vi "Eval_SglVar_SglRes.vi"(8 "error in (no error)":errorcluster, 9 "varValue":dbl format="%#_13g", 11 "mupExpr in":refnum<data-value>) -> (0 "error out":errorcluster, 2 "Result":dbl, 3 "mupExpr out":refnum<data-value>)   [LabVIEW 2015, in "mupExpr.lvclass"]
doc: "Updates the value of the selected single variable then evaluates the expression.\nReturns a single result.\n\nIf multiple expressions have been input, the result of the last one in the list is returned.\n\nIf the variables are defined for bulk mode evaluation, only the first set (index 0) will be evaluated."
uses:
  mupExpr.lvclass
  mupExpr.lvclass/mupExpr.ctl
  mupLib/mupCheckError.vi
  mupLib/mupLibPath.vi
  <vilib>/Utility/error.llb/Error Cluster From Error Code.vi
  mupLib/mupLib.lvlib
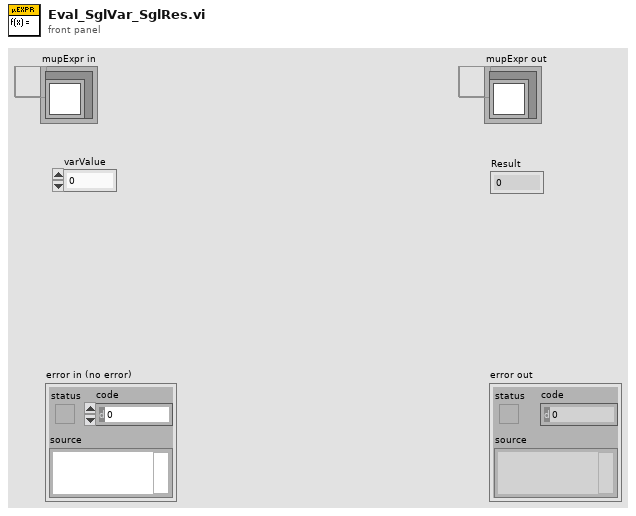
[diagram p1: front panel]
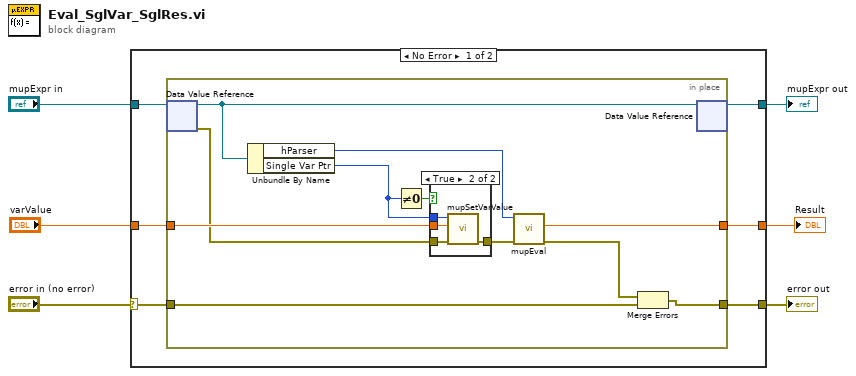
[diagram p0: block diagram]
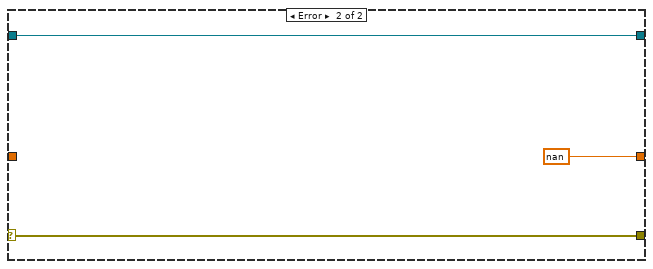
[diagram p3: hidden frame]
diagram:
  n1 = case shown="No Error" "error in (no error)" {
    selector: "error in (no error)" -> [w12 w31]
    tunnel: [w10 w31] -> w5
    tunnel: [w7 w30] -> w3
    tunnel: "mupExpr in" -> [w8 w30]
    tunnel: "varValue" -> [w11 _]
    tunnel: [w9 nan ("Result")] -> w1
    frame No Error {
      n2 = in-place {
        in-place-border: w12 -> [w17]
        in-place-border: w11 -> [w22]
        in-place-border: [w15] -> w10
        in-place-border: [w21] -> w9
        n3 = in-place-dvr #1(w8) -> (w18:refnum<class "mupExpr.lvclass">, w19:errorcluster)
        n4 = Unbundle By Name(w18) -> ("hParser"=w20:u64, "Single Var Ptr"=w23:u64)
        n5 = Not Equal To 0?(x=w23) -> (x != 0?=w13:bool)
        n6 = case shown="True" w13 {
          tunnel: w19 -> [w24 w28]
          tunnel: w22 -> [_ w27]
          tunnel: [w24 w26] -> w14
          tunnel: w23 -> [_ w25]
          frame False {
          }
          frame True {
            n7 = call "mupSetVarValue.vi"("error in (no error)"=w28, "varValue"=w27, "varAddr in"=w25) -> ("error out"=w26:errorcluster)  [unwired: 7 in, 1 out]
          }
        }
        n8 = call "mupEval.vi"("error in (no error)"=w14, "hParser in"=w20) -> ("error out"=w16:errorcluster, "result"=w21:dbl)  [unwired: 7 in, 1 out]
        n9 = Merge Errors(w16, w17) -> (w15:errorcluster)
        n10 = in-place-dvr #1(w18) -> (w7:refnum<data-value>)  [unwired: 1 out]
      }
    }
    frame Error {
    }
  }
  "error out" <- w5
  "mupExpr out" <- w3
  "Result" <- w1
